vi "Config_HD_Write.vi"() -> ()   [LabVIEW 2016]
uses:
  MW_ctl_DeviceHandles..ctl
  <vilib>/Utility/config.llb/Write Key (String).vi
  Microwave Source.lvlib
  <vilib>/Utility/config.llb/NI_LVConfig.lvlib
panel:
  out "HardwareAddress.ini":path
  out "error out":errorcluster
  in  "error in (no error)":errorcluster
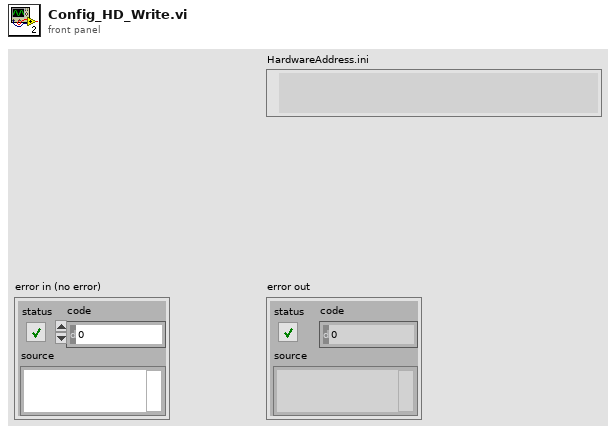
[diagram p1: front panel]
types:
  T1 = typedef "Microwave Source.lvlib/MW_ctl_DeviceHandles..ctl" = cluster{"LO VISA":refnum<visa-resource-name>, "Probe VISA":refnum<visa-resource-name>, "Qubits":refnum<visa-resource-name>[]}
  T2 = typedef "Constant_FilePaths_ctl.ctl" = cluster{"Directories":cluster{"Application":path, "Config":path}, "Files":cluster{"HardwareAddress.ini":path}}
  T3 = typedef "NI_LVConfig.lvlib/Config Data RefNum.ctl" = refnum<k1>
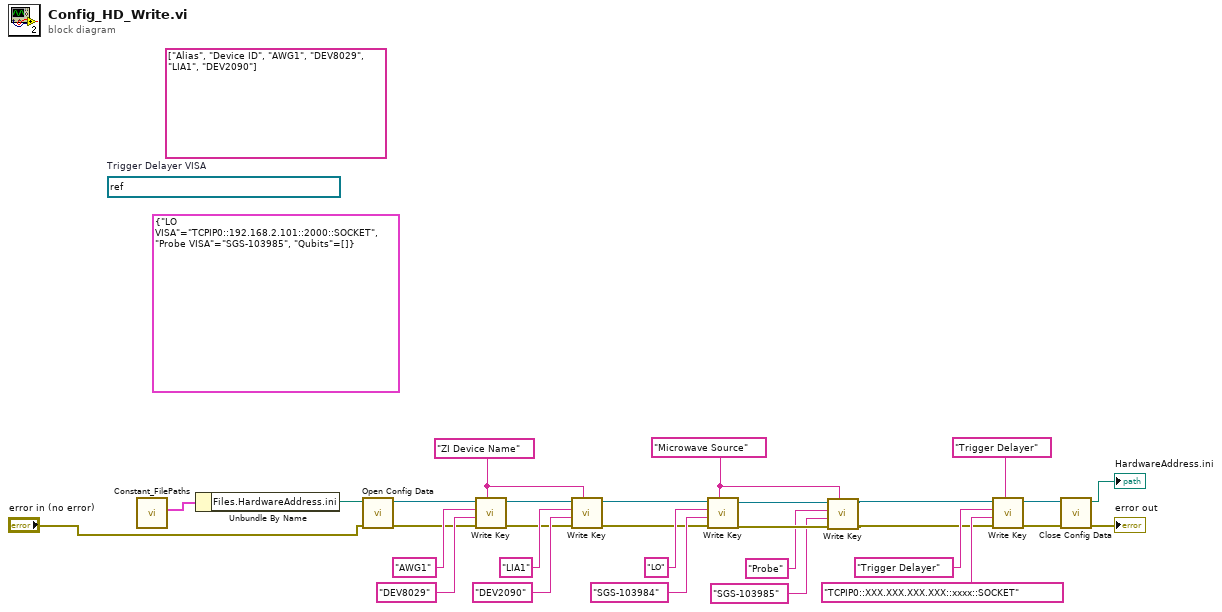
[diagram p0: block diagram]
diagram:
  w23 = "Microwave Source" ("section")
  w24 = "ZI Device Name" ("section")
  (unwired) refnum<visa-resource-name> "TCPIP0::192.168.2.10::5025::SOCKET"  # Trigger Delayer VISA
  (unwired) T1 {"LO VISA"="TCPIP0::192.168.2.101::2000::SOCKET", "Probe VISA"="SGS-103985", "Qubits"=[]} ("MW Source In")
  (unwired) string[][] [["Alias", "Device ID"], ["AWG1", "DEV8029"], ["LIA1", "DEV2090"]] ("Hardware Handle.Device Name")
  n1 = call "Constant_FilePaths.vi"() -> ("Paths"=w5:T2)  [unwired: 11 in]
  n2 = Unbundle By Name(w5) -> ("Files.HardwareAddress.ini"=w4:path)
  n3 = call <vilib>:"Open Config Data.vi"("error in (no error)"="error in (no error)", "configuration file path"=w4) -> ("error out"=w13:errorcluster, "refnum"=w14:T3)  [unwired: 7 in, 1 out]
  n4 = call-poly <vilib>:"Write Key.vi"("section"=w24, "error in (no error)"=w13, "value"="DEV8029" ("key"), "key"="AWG1", "refnum"=w14) -> ("error out"=w26:errorcluster, "refnum out"=w25:T3)  [unwired: 4 in, 1 out]
  n5 = call-poly <vilib>:"Write Key.vi"("section"=w24, "error in (no error)"=w26, "value"="DEV2090" ("key"), "key"="LIA1", "refnum"=w25) -> ("error out"=w15:errorcluster, "refnum out"=w16:T3)  [unwired: 4 in, 1 out]
  n6 = call-poly <vilib>:"Write Key.vi"("section"=w23, "error in (no error)"=w15, "value"="SGS-103984" ("key"), "key"="LO", "refnum"=w16) -> ("error out"=w21:errorcluster, "refnum out"=w22:T3)  [unwired: 4 in, 1 out]
  n7 = call-poly <vilib>:"Write Key.vi"("section"=w23, "error in (no error)"=w21, "value"="SGS-103985" ("key"), "key"="Probe", "refnum"=w22) -> ("error out"=w9:errorcluster, "refnum out"=w10:T3)  [unwired: 4 in, 1 out]
  n8 = call-poly <vilib>:"Write Key.vi"("section"="Trigger Delayer", "error in (no error)"=w9, "value"="TCPIP0::XXX.XXX.XXX.XXX::xxxx::SOCKET" ("key"), "key"="Trigger Delayer", "refnum"=w10) -> ("error out"=w8:errorcluster, "refnum out"=w7:T3)  [unwired: 4 in, 1 out]
  n9 = call <vilib>:"Close Config Data.vi"("error in (no error)"=w8, "refnum"=w7) -> ("error out"=→"error out":errorcluster, "file path"=→"HardwareAddress.ini":path)  [unwired: 8 in]
